vi "PDSS - Trigger Sequence - Calculate 2kHz Waveform.vi"(8 "error in":errorcluster, 10 "Time (200 ms)":dbl=200.0, 11 "Voltages":dbl[](array[numeric])=[1.0, 1.1, 1.2000000000000002, 1.3000000000000003] format="%.3g") -> (0 "error out":errorcluster, 3 "tuning waveforms":waveform(dbl)[](array[waveform])=[{"t0"=timestamp(0 s since 1904-01-01), "dt"=0.000125, "Y"=array[1600 elements]}, {"t0"=timestamp(0 s since 1904-01-01), "dt"=0.000125, "Y"=array[1600 elements]}, {"t0"=timestamp(0 s since 1904-01-01), "dt"=0.000125, "Y"=array[1600 elements]}, {"t0"=timestamp(0 s since 1904-01-01), "dt"=0.000125, "Y"=array[1600 elements]}])   [LabVIEW 2014]
doc: "This VI generates the analog waveforms necessary to tune the Lyot filter to a particular wavelength. The wavelength is controlled by the 2kHz AC (0-10 Vrms) analog voltages applied to each of 4 nematic liquid crystals from Meadowlark Optics.\n\nThe sampling information for this VI is generated externally in the calling VI which generates the polarization modulation waveforms applied to the FLC liquid crystals."
uses:
  <vilib>/measure/NI_MABase.lvlib
panel:
  out "Waveform Graph":waveform(dbl)[](graph)=[{"t0"=timestamp(0 s since 1904-01-01), "dt"=0.000125, "Y"=array[1600 elements]}, {"t0"=timestamp(0 s since 1904-01-01), "dt"=0.000125, "Y"=array[1600 elements]}, {"t0"=timestamp(0 s since 1904-01-01), "dt"=0.000125, "Y"=array[1600 elements]}, {"t0"=timestamp(0 s since 1904-01-01), "dt"=0.000125, "Y"=array[1600 elements]}]
  # "Nematic LC's require a modulation frequency of 2 kHz.  \n\nFor a 2kHz waveform defined by 4 points per cycle, \nwe need a 8000 AO points per second sampling Frequency (Fs).  This means the hardsware\nupdates DAQ voltages every 125 microseconds.   \n\nA single LCVR modulation cycle (4 points) requires 500 microseconds.\n\nA 0.2 seconds modulation requires 1600 point (0.2 / 0.000125)\n\nMatus and Scott selected 0.2 seconds because this is equal to the relaxation time\nof the LCVR's and creates a nice 'brick' for constructing long series of voltages"
  # "Liquid Crystal Variable Retarders"
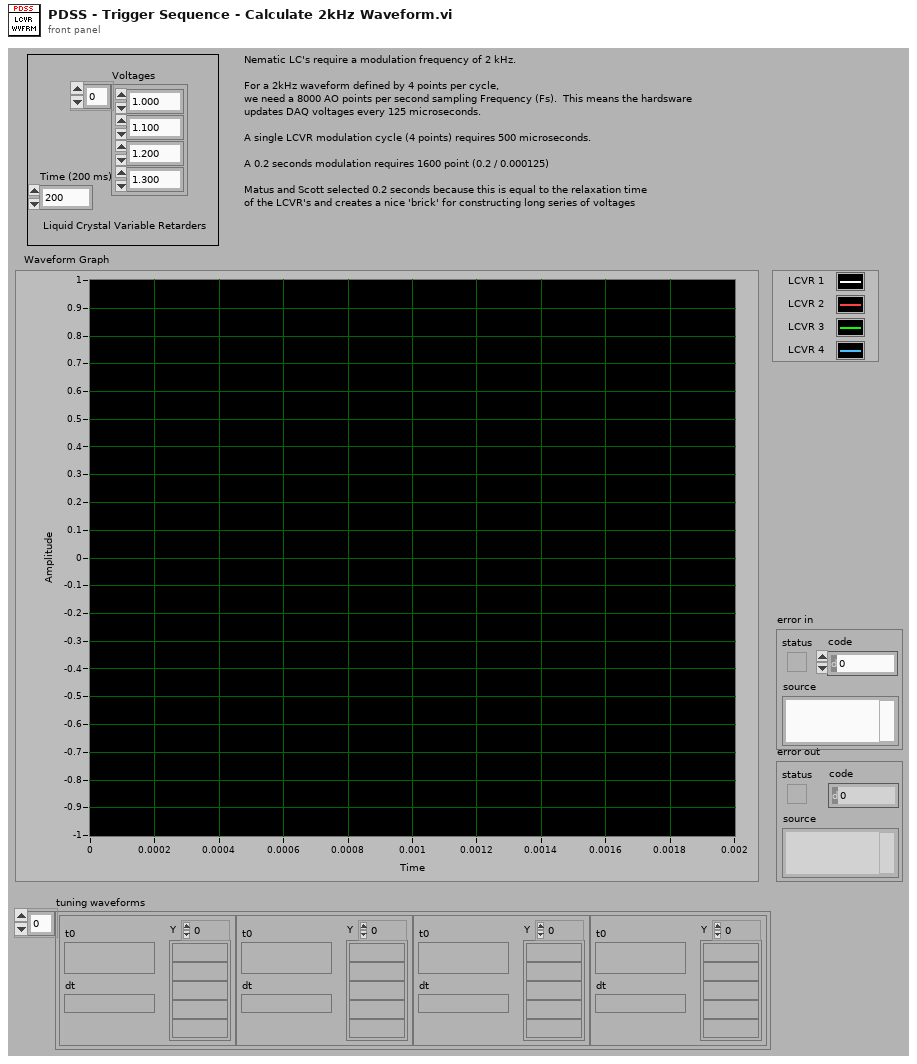
[diagram p1: front panel]
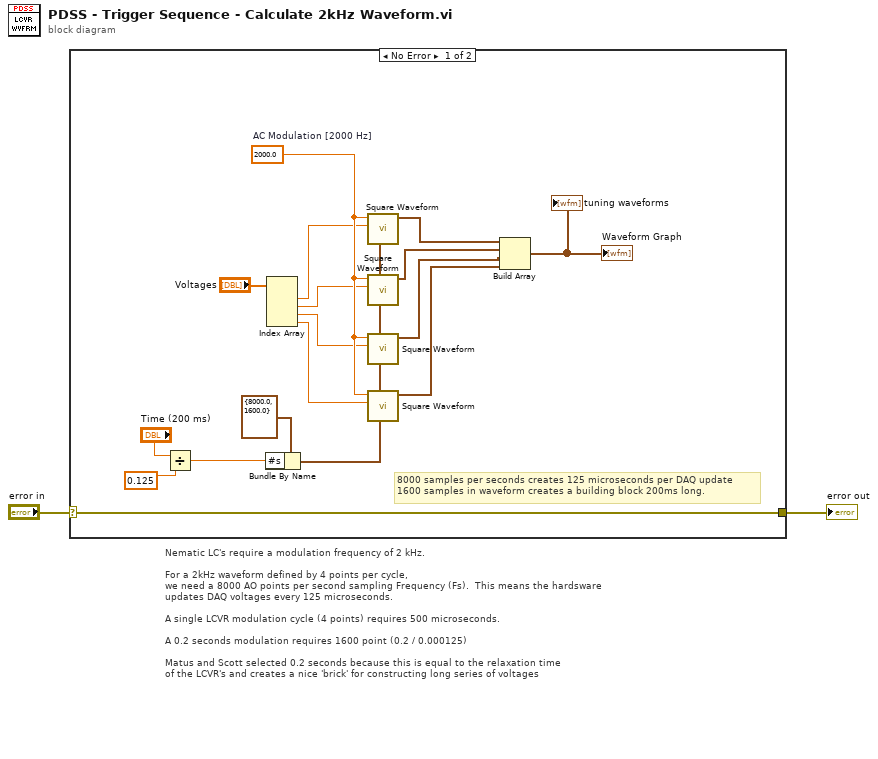
[diagram p0: block diagram]
diagram:
  # "Nematic LC's require a modulation frequency of 2 kHz.  \n\nFor a 2kHz waveform defined by 4 points per cycle, \nwe need a 8000 AO points per second sampling Frequency (Fs).  This means the hardsware\nupdates DAQ voltages every 125 microseconds.   \n\nA single LCVR modulation cycle (4 points) requires 500 microseconds.\n\nA 0.2 seconds modulation requires 1600 point (0.2 / 0.000125)\n\nMatus and Scott selected 0.2 seconds because this is equal to the relaxation time\nof the LCVR's and creates a nice 'brick' for constructing long series of voltages"
  n1 = case shown="No Error" "error in" {
    selector: "error in" -> [w19 w20]
    tunnel: [w19 w20] -> w1
    frame No Error {
      w12 = 2000.0  # AC Modulation [2000 Hz]
      # "8000 samples per seconds creates 125 microseconds per DAQ update\n1600 samples in waveform creates a building block 200ms long."
      n2 = Divide(x="Time (200 ms)", y=0.125) -> (x/y=w3:dbl)
      n3 = Bundle By Name(cluster=cluster{"Fs":dbl, "#s":dbl} {"Fs"=8000.0, "#s"=1600.0} ("sampling info"), "#s"=w3) -> (w7:cluster{"Fs":dbl, "#s":dbl})
      n4 = Index Array(array="Voltages") -> (element #1=w11:dbl, element #2=w10:dbl, element #3=w9:dbl, element #4=w8:dbl)  [unwired: 4 in]
      n5 = call <vilib>:"Square Waveform.vi"("sampling info"=w7, "amplitude"=w11, "frequency"=w12) -> ("signal out"=w17:waveform(dbl))  [unwired: 7 in, 1 out]
      n6 = call <vilib>:"Square Waveform.vi"("sampling info"=w7, "amplitude"=w10, "frequency"=w12) -> ("signal out"=w16:waveform(dbl))  [unwired: 7 in, 1 out]
      n7 = call <vilib>:"Square Waveform.vi"("sampling info"=w7, "amplitude"=w9, "frequency"=w12) -> ("signal out"=w15:waveform(dbl))  [unwired: 7 in, 1 out]
      n8 = call <vilib>:"Square Waveform.vi"("sampling info"=w7, "amplitude"=w8, "frequency"=w12) -> ("signal out"=w14:waveform(dbl))  [unwired: 7 in, 1 out]
      n9 = Build Array(w17, w16, w15, w14) -> (→"Waveform Graph" →"tuning waveforms":waveform(dbl)[])
    }
    frame Error {
    }
  }
  "error out" <- w1
